vi "Module Name--constant.vi"() -> (3 "Module Name":string="Chart Module")   [LabVIEW 2014, in "Chart Module.lvlib"]
uses:
  Chart Module.lvlib
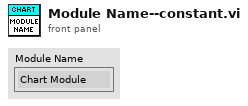
[diagram p1: front panel]
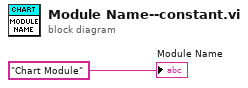
[diagram p0: block diagram]
diagram:
  "Module Name" <- "Chart Module"
